vi "Layout - Five.vi"(4 "Section 5":string, 5 "Width (1800)":i32=1800, 6 "Section 4":string, 8 "Error in":errorcluster caption="Error in (no error)", 9 "Section 3":string, 10 "Section 2":string, 11 "Section 1":string) -> (0 "Error out":errorcluster, 3 "Text Output":string)   [LabVIEW 2023, in "Confluence Formatting.lvlib"]
uses:
  Confluence Formatting.lvlib
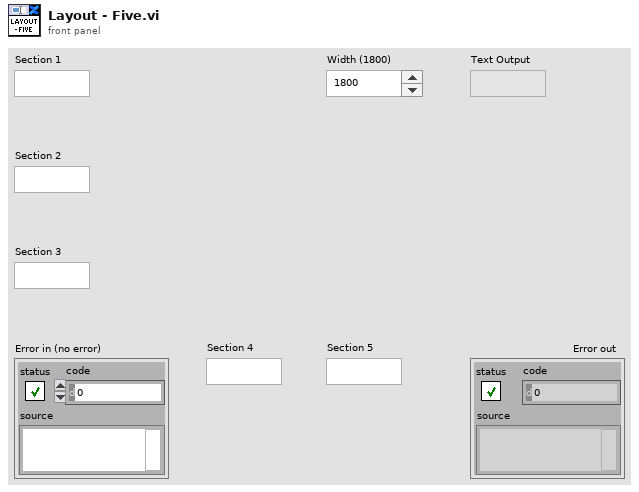
[diagram p1: front panel]
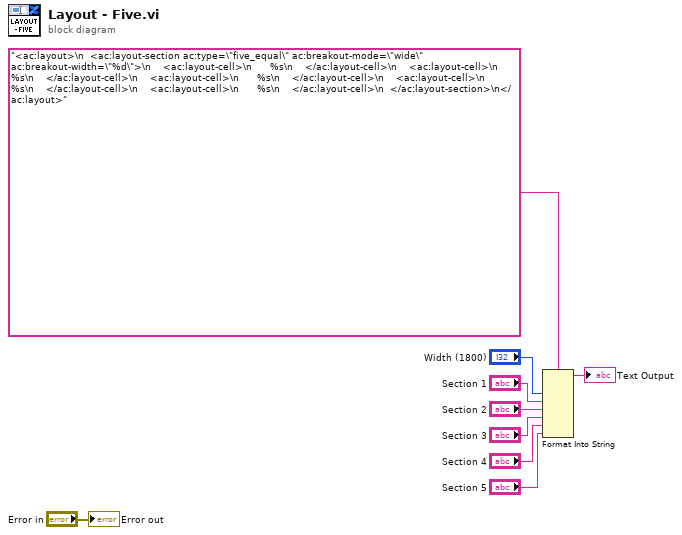
[diagram p0: block diagram]
diagram:
  n1 = Format Into String(format string="<ac:layout>\n  <ac:layout-section ac:type=\"five_equal\" ac:breakout-mode=\"wide\" ac:breakout-width=\"%d\">\n    <ac:layout-cell>\n      %s\n    </ac:layout-cell>\n    <ac:layout-cell>\n      %s\n    </ac:layout-cell>\n    <ac:layout-cell>\n      %s\n    </ac:layout-cell>\n    <ac:layout-cell>\n      %s\n    </ac:layout-cell>\n    <ac:layout-cell>\n      %s\n    </ac:layout-cell>\n  </ac:layout-section>\n</ac:layout>", "Width (1800)", "Section 1", "Section 2", "Section 3", "Section 4", "Section 5") -> (resulting string=→"Text Output":string)  [unwired: 2 in, 1 out]
  "Error out" <- "Error in"
